vi "SPI Host.vi"() -> ()   [LabVIEW 2012]
uses:
  <vilib>/FPGAPlugInAG/sbRIO-9636/niLvFpga_Open_sbRIO-9636.vi
  <vilib>/rvi/interface/common/dynamic/niFpgaDynamicAddResources.vi
  <vilib>/FPGAPlugInAG/Dynamic/niLvFpga_Close_Dynamic.vi
  <vilib>/rvi/interface/nirviOpenFPGA/nirviOpenFPGA.xnode
  FPGA Bitfiles/NIARC_FPGATarget_SPIFPGA_Wqb9KPQaEsk.lvbitx
  FPGA/SPI FPGA.vi
  <vilib>/rvi/interface/nirviCloseFPGA/nirviCloseFPGA.xnode
  <vilib>/IEDriver/SPIandI2C/Host/SPI/SPI Host.lvlib
panel:
  in  "Write?":bool
  in  "stop":bool
  in  "Write Data":u8[](array[numeric])=[49, 11, 45, 8, 46, 128] format="%.0x"
  out "Read Data":u8[](array[numeric])
  in  "CS Active State":bool
  in  "Timeout (10 s)":u8=10
  in  "FPGA Clock (40 MHz)":u32=40000000
  in  "Port Number":u8
  in  "Number of Bits":u16=16
  in  "Chip Select":T1(ring)
  in  "Clock Rate":u32=100
  in  "Mode":u8=3
  # "This example demonstrates how to use SPI driver to communicate with SPI device.\nThis example is intentionally broken until you compile this example for a specific target."
  # "Configuration"
  # "Write & Read"
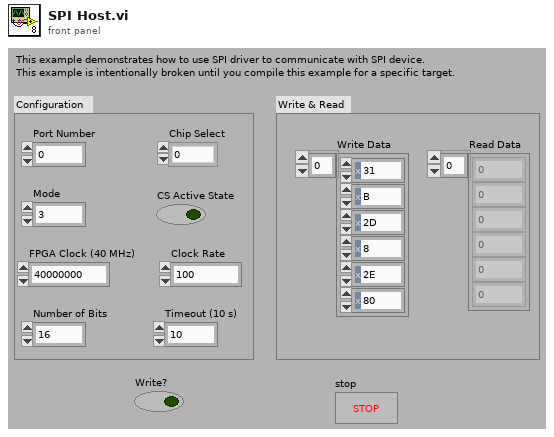
[diagram p1: front panel]
types:
  T1 = enum16{"0", "1", "2", "3", "4", "5", "6", "7", "8", "9"}
  T2 = cluster{"FPGA VI Reference":refnum<k20>, "Port Number":u8}
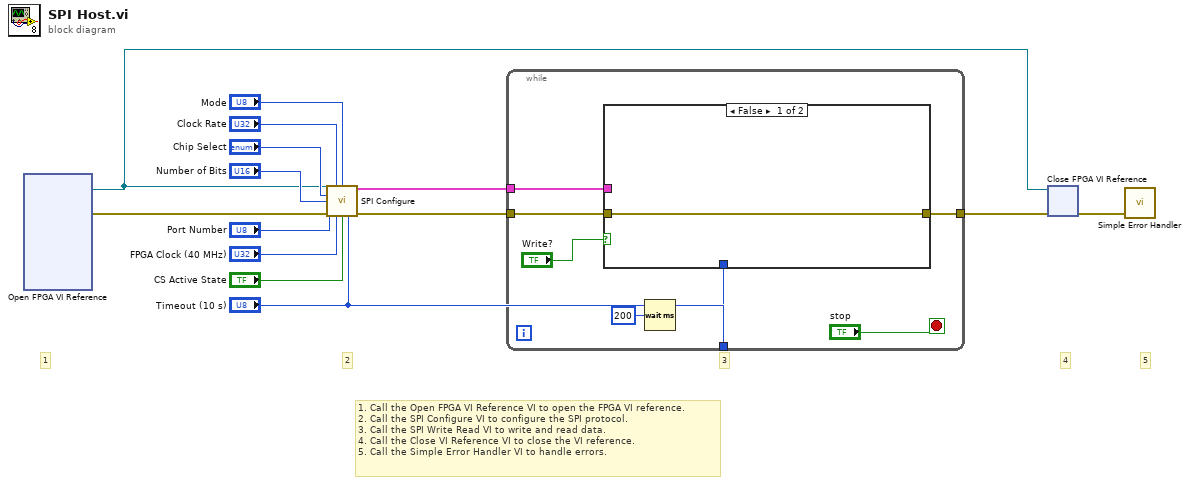
[diagram p0: block diagram]
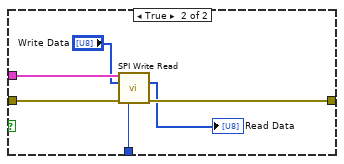
[diagram p2: hidden frame]
diagram:
  # "5"
  # "4"
  # "3"
  # "2"
  # "1"
  # "1. Call the Open FPGA VI Reference VI to open the FPGA VI reference.\n2. Call the SPI Configure VI to configure the SPI protocol.\n3. Call the SPI Write Read VI to write and read data.\n4. Call the Close VI Reference VI to close the VI reference.\n5. Call the Simple Error Handler VI to handle errors."
  n1 = xnode "Open FPGA VI Reference"() -> ("FPGA VI Reference Out"=w2:refnum<k20>, "error out"=w1:errorcluster)  [unwired: 2 in]
  n2 = call <vilib>:"SPI Configure.vi"("FPGA VI Reference"=w2, "Clock Rate"="Clock Rate", "Mode"="Mode", "Chip Select"="Chip Select", "Number of Bits"="Number of Bits", "Port Number"="Port Number", "error in (no error)"=w1, "FPGA Clock (40 MHz)"="FPGA Clock (40 MHz)", "CS Active State"="CS Active State", "Timeout (10 s)"="Timeout (10 s)") -> ("FPGA Information Out"=w13:T2, "error out"=w14:errorcluster)  [unwired: 4 in]
  n3 = while {
    tunnel: w14 -> [w21]
    tunnel: w13 -> [w20]
    tunnel: [w19] -> w12
    tunnel: "Timeout (10 s)" -> [w18]
    stop <- "stop" stop-if-true
    n4 = case shown="False" "Write?" {
      tunnel: w21 -> [w22 w28]
      tunnel: w20 -> [_ w27]
      tunnel: [w22 w26] -> w19
      tunnel: w18 -> [_ w25]
      frame False {
      }
      frame True {
        n5 = call <vilib>:"SPI Write Read.vi"("FPGA Information In"=w27, "Write Data"="Write Data", "error in (no error)"=w28, "Timeout (10 s)"=w25) -> ("Read Data"=→"Read Data":u8[], "error out"=w26:errorcluster)  [unwired: 9 in, 1 out]
      }
    }
    n6 = Wait (ms)(milliseconds to wait=u32 200) -> ()  [unwired: 1 out]
  }
  n7 = xnode "Close FPGA VI Reference"("FPGA VI Reference In"=w2, "error in"=w12) -> ("error out"=w3:errorcluster)
  n8 = call <vilib>:"Simple Error Handler.vi"("error in (no error)"=w3) -> ()  [unwired: 4 in, 5 out]
